vi "Main.vi"() -> ()   [LabVIEW 2013]
uses:
  <vilib>/myRIO/Instrument Drivers/Onboard IO/I2C/typedefs/I2C User Configuration.ctl
  <vilib>/myRIO/Instrument Drivers/Onboard IO/I2C/typedefs/I2C Transfer Rate.ctl
  <vilib>/Platform/TimedLoop/XDataNode/timing_clust.ctl
  <vilib>/Platform/TimedLoop/XDataNode/nitl_modes.ctl
  <vilib>/Platform/TimedLoop/XDataNode/wakeup.ctl
  <vilib>/myRIO/Common/Instrument Driver Framework/myRIO v1.0/I2C/vis/myRIO v1.1 Open I2C.vi
  <vilib>/myRIO/Common/Instrument Driver Framework/myRIO v1.0/UART/vis/myRIO v1.0 Close UART.vi
  <vilib>/myRIO/Common/Instrument Driver Framework/Utilities/vis/Validate Channels.vi
  <vilib>/myRIO/Common/Instrument Driver Framework/myRIO v1.0/I2C/vis/myRIO v1.0 Reserve I2C.vi
  <vilib>/myRIO/Common/Instrument Driver Framework/myRIO v1.0/I2C/vis/myRIO v1.0 Build MUX Configuration I2C.vi
  <vilib>/myRIO/Common/Instrument Driver Framework/myRIO v1.0/Resource Manager/vis/myRIO v1.0 Reserve Channel List.vi
  <vilib>/myRIO/Common/Instrument Driver Framework/myRIO v1.0/Resource Manager/vis/myRIO v1.0 Create Configuration List.vi
  <vilib>/myRIO/Common/Instrument Driver Framework/myRIO v1.0/Resource Manager/vis/myRIO v1.0 Reserve Channel.vi
  <vilib>/myRIO/Common/Instrument Driver Framework/myRIO v1.0/Resource Manager/vis/myRIO v1.0 Unreserve Channel.vi
  <vilib>/myRIO/Common/Instrument Driver Framework/myRIO v1.0/Resource Manager/vis/myRIO v1.0 Build Mutex Name.vi
  <vilib>/myRIO/Common/Instrument Driver Framework/myRIO v1.0/myRIO v1.1 Open.vi
  <vilib>/Utility/VariantDataType/GetNumericInfo.vi
  <vilib>/Utility/error.llb/Error Cluster From Error Code.vi
  <vilib>/myRIO/Common/Instrument Driver Framework/Utilities/vis/IO Manager.vi
  <vilib>/myRIO/Common/Instrument Driver Framework/Utilities/vis/Configuration Manager.vi
  <vilib>/myRIO/Common/Instrument Driver Framework/myRIO v1.0/Resource Manager/vis/myRIO v1.0 Configure IO.vi
  <vilib>/myRIO/Common/Instrument Driver Framework/myRIO v1.0/myRIO v1.0 Close.vi
  <vilib>/myRIO/Common/Instrument Driver Framework/myRIO v1.0/I2C/vis/myRIO v1.0 Configure I2C.vi
  <vilib>/myRIO/Common/Instrument Driver Framework/myRIO v1.0/I2C/vis/myRIO v1.0 Write I2C.vi
  <vilib>/myRIO/Common/Instrument Driver Framework/myRIO v1.0/I2C/vis/myRIO v1.0 Read I2C.vi
  <vilib>/myRIO/Common/Instrument Driver Framework/Utilities/vis/FPGA Ref Manager.vi
  <vilib>/myRIO/Common/Instrument Driver Framework/myRIO v1.0/myRIO v1.0 Reset FPGA.vi
  <vilib>/platform/TimedLoop/XDataNode/XDataNode.xnode
  <vilib>/myRIO/Instrument Drivers/Utilities/Utilities.lvlib
  <vilib>/myRIO/Instrument Drivers/Onboard IO/I2C/I2C.lvlib
  <vilib>/Platform/TimedLoop/XDataNode/XDNodeRunTimeDep.lvlib
panel:
  out "X rate":i16
  out "Y rate":i16
  out "Z rate":i16
  out "Gyroscope: Angular rate [LSB/sec]":cluster{i16, i16, i16}(graph)
  out "Accelerometer: Waveform Chart":cluster{i16, i16, i16}(graph)
  out "Z":i16
  out "Y":i16
  out "X":i16
  in  "[ESC]":bool
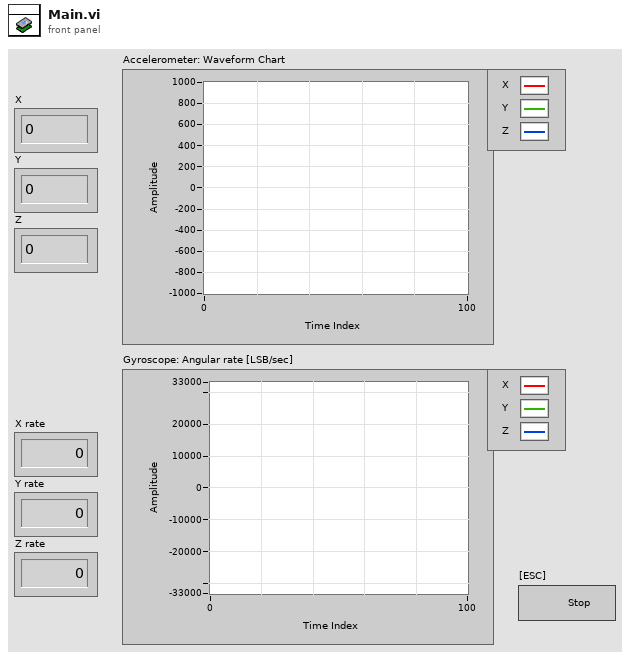
[diagram p1: front panel]
types:
  T1 = typedef "I2C.lvlib/I2C User Configuration.ctl" = cluster{"I2C Transfer Rate":T2}
  T2 = typedef "I2C.lvlib/I2C Transfer Rate.ctl" = enum16{"Standard Mode (100 kbps)", "Fast Mode (400 kbps)"}
  T3 = typedef "I2C.lvlib/I2C Reference.ctl" = cluster{"myRIO Reference":T4, "I2C Channels Enum":T8, "I2C Configuration":T9}
  T4 = typedef "myRIO Generic Hardware Reference.ctl" = cluster{"myRIO Model":T5, "myRIO Hardware Reference":T6}
  T5 = typedef "Hardware Version Enum.ctl" = enum16{"Unknown", "myRIO-1900", "myRIO-1950"}
  T6 = typedef "myRIO v1.0 Reference.ctl" = cluster{"Generic FPGA Reference":T7, "Allow multiple opens":bool}
  T7 = typedef "Generic FPGA Reference.ctl" = refnum<k20>
  T8 = typedef "I2C Channels Enum.ctl" = enum16{"Not Connected", "A/I2C", "B/I2C"}
  T9 = typedef "I2C.lvlib/I2C Configuration.ctl" = cluster{"I2C Transfer Rate":T2}
  T10 = typedef "XDNodeRunTimeDep.lvlib/timing_clust.ctl" = cluster{"Expected End [f-1]":u64, "Actual End [f-1]":u64, "Finished Late? [f-1]":bool, "Expected End [i-1]":u64, "Actual End [i-1]":u64, "Finished Late? [i-1]":bool, "Expected Start [i]":u64, "Actual Start [i]":u64, "Expected Start [f]":u64, "Actual Start [f]":u64, "Source Name":string, "Structure Name":string, "Period":i64, "Deadline":i64, "Offset":i64, "Start":i64, "Priority":i32, "Timeout":i32, "Mode":T11, "Wakeup Reason":T12, "Error":errorcluster, "Source Type":string, "Secondary Source Type":string, "Global End Time":u64, "Global Start Time":u64, "Frame Duration":u64, "Iteration Duration":u64, "Assigned CPU":i32, "I/O Scan Engine Mode":u32}
  T11 = typedef "XDNodeRunTimeDep.lvlib/nitl_modes.ctl" = enum32{"No Change", "Process missed periods, maintain original phase", "Discard missed periods, maintain original phase", "Process missed periods, ignore original phase", "Discard missed periods, ignore original phase"}
  T12 = typedef "XDNodeRunTimeDep.lvlib/wakeup.ctl" = enum32{"Normal", "Aborted", "Asynchronous wakeup", "Timing source error", "Timed loop error", "Timeout"}
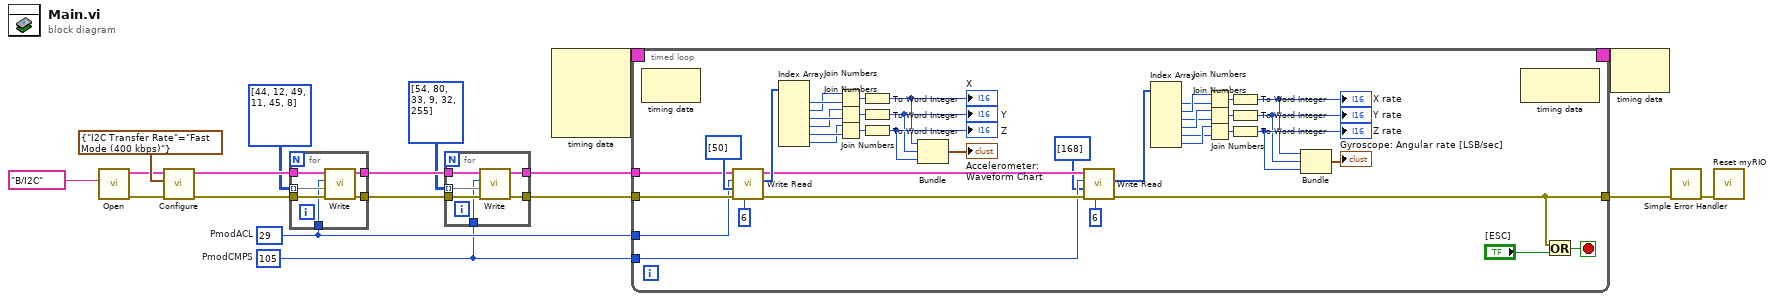
[diagram p0: block diagram]
diagram:
  w2 = u8 105  # PmodCMPS
  w3 = u8 29  # PmodACL
  n1 = call <vilib>:"Open.vi"("Channel Name"=tag "B/I2C" ("I2C channel")) -> ("error out"=w14:errorcluster, "I2C Ref Out"=w15:T3)  [unwired: 9 in]
  n2 = call <vilib>:"Configure.vi"("error in (no error)"=w14, "I2C User Configuration"=T1 {"I2C Transfer Rate"=enum."Fast Mode (400 kbps)"} ("I2C bus speed"), "I2C Ref In"=w15) -> ("error out"=w12:errorcluster, "I2C Ref Out"=w13:T3)  [unwired: 7 in]
  n3 = for {
    tunnel: [w24] -> w4
    tunnel: [w23] -> w5
    tunnel: u8[][] [[44, 12], [49, 11], [45, 8]] ("Bytes to Write") -> [w22] mode=indexing
    tunnel: w13 -> [w21]
    tunnel: w12 -> [w20]
    tunnel: w3 -> [w19]
    n4 = call <vilib>:"Write.vi"("error in (no error)"=w20, "Bytes to Write"=w22, "Slave Address (7-bit)"=w19, "I2C Ref In"=w21) -> ("error out"=w24:errorcluster, "I2C Ref Out"=w23:T3)  [unwired: 6 in]
  }
  n5 = for {
    tunnel: [w30] -> w6
    tunnel: [w29] -> w7
    tunnel: u8[][] [[54, 80], [33, 9], [32, 255]] ("Bytes to Write") -> [w28] mode=indexing
    tunnel: w5 -> [w27]
    tunnel: w4 -> [w26]
    tunnel: w2 -> [w25]
    n6 = call <vilib>:"Write.vi"("error in (no error)"=w26, "Bytes to Write"=w28, "Slave Address (7-bit)"=w25, "I2C Ref In"=w27) -> ("error out"=w30:errorcluster, "I2C Ref Out"=w29:T3)  [unwired: 6 in]
  }
  n7 = node-c288() -> (w11:T10)  [unwired: 4 in]
  n8 = timed-loop {
    tunnel: w6 -> [w52]
    tunnel: w7 -> [w53]
    timing: w11 -> [_]
    timing-out: [_] -> w10
    tunnel: [w45] -> w8
    tunnel: w3 -> [w51]
    tunnel: w2 -> [w47]
    stop <- w71 stop-if-true
    n9 = node-c288() -> ()  [unwired: 1 in, 1 out]
    n10 = call <vilib>:"Write Read.vi"("Byte Count"=u32 6, "error in (no error)"=w52, "Bytes to Write"=u8[] [50], "Slave Address (7-bit)"=w51, "I2C Ref In"=w53) -> ("error out"=w48:errorcluster, "Bytes Read"=w54:u8[], "I2C Ref Out"=w49:T3)  [unwired: 3 in]
    n11 = Index Array(array=w54) -> (element #1=w62:u8, element #2=w61:u8, element #3=w60:u8, element #4=w59:u8, element #5=w58:u8, element #6=w57:u8)  [unwired: 6 in]
    n12 = Join Numbers(hi=w61, lo=w62) -> ((hi.lo)=w69:u16)
    n13 = Join Numbers(hi=w59, lo=w60) -> ((hi.lo)=w68:u16)
    n14 = Join Numbers(hi=w57, lo=w58) -> ((hi.lo)=w67:u16)
    n15 = To Word Integer(number=w69) -> (16bit integer=w64:i16)
    "X" <- w64
    n16 = To Word Integer(number=w68) -> (16bit integer=w63:i16)
    "Y" <- w63
    n17 = To Word Integer(number=w67) -> (16bit integer=w66:i16)
    "Z" <- w66
    n18 = Bundle(w64, w63, w66) -> (→"Accelerometer: Waveform Chart":cluster{i16, i16, i16})  [unwired: 1 in]
    n19 = call <vilib>:"Write Read.vi"("Byte Count"=u32 6, "error in (no error)"=w48, "Bytes to Write"=u8[] [168], "Slave Address (7-bit)"=w47, "I2C Ref In"=w49) -> ("error out"=w45:errorcluster, "Bytes Read"=w31:u8[])  [unwired: 3 in, 1 out]
    n20 = Index Array(array=w31) -> (element #1=w36:u8, element #2=w37:u8, element #3=w38:u8, element #4=w39:u8, element #5=w40:u8, element #6=w41:u8)  [unwired: 6 in]
    n21 = Join Numbers(hi=w37, lo=w36) -> ((hi.lo)=w32:u16)
    n22 = Join Numbers(hi=w39, lo=w38) -> ((hi.lo)=w33:u16)
    n23 = Join Numbers(hi=w41, lo=w40) -> ((hi.lo)=w34:u16)
    n24 = To Word Integer(number=w32) -> (16bit integer=w42:i16)
    "X rate" <- w42
    n25 = To Word Integer(number=w33) -> (16bit integer=w43:i16)
    "Y rate" <- w43
    n26 = To Word Integer(number=w34) -> (16bit integer=w44:i16)
    "Z rate" <- w44
    n27 = Bundle(w42, w43, w44) -> (→"Gyroscope: Angular rate [LSB/sec]":cluster{i16, i16, i16})  [unwired: 1 in]
    n28 = node-c288() -> ()  [unwired: 1 in, 1 out]
    n29 = Or(x=w45, y="[ESC]") -> (x .or. y?=w71:bool)
  }
  n30 = node-c288(w10) -> ()  [unwired: 1 out]
  n31 = call <vilib>:"Simple Error Handler.vi"("error in (no error)"=w8) -> ("error out"=w18:errorcluster)  [unwired: 4 in, 4 out]
  n32 = call <vilib>:"Reset myRIO.vi"("error in (no error)"=w18) -> ()  [unwired: 10 in, 1 out]
